vi "Close.vi"(8 "error in (no error)":errorcluster, 11 "State Variables in":T1={"NIVS.CachedDataRef"=refnum, "NIVS.LaunchRef"=refnum, "NIVS.SysDefRoot"=refnum, "NIVS.Workspace"=refnum, "NIVS.CachedData"={"Name"="", "Node Path"="", "Caption"="", "List"={"AutoUpdate"=FALSE, "Names"=[], "Values"=[], "Symbols"=[]}}, "NIVS.SystemStateRefs"={"CustDatRef"=refnum, "EvtRef"=refnum, "Target State User Event"=refnum}, "NIVS.UserEventRefs"={"SystemChangeEventRef"=refnum, "Event Registration Refnum"=refnum}, "Workspace.Connected?"=FALSE, "Workspace.ChannelFound?"=FALSE, "UI.Listbox"=refnum, "VS.DisplayFilter"=7, "Force?"=FALSE} {"VS.DisplayFilter" items=["K_CHAN_R", "K_CHAN_W", "K_CHAN_RW", "K_CHAN_VOLT", "K_CHAN_FAULT", "K_ALL", "K_CUSTOM", "K_CHAN_R_VIS", "K_CHAN_W_VIS", "K_CHAN_RW_VIS", "K_CHAN_VOLT_VIS", "K_CHAN_FAULT_VIS"]}) -> ()   [LabVIEW 2015, in "Workspace.Obejct.Radio.lvlib"]
uses:
  Workspace.Obejct.Radio.lvlib
  Types/StateVariables.ctl
  <vilib>/NI Veristand/Display Template Support/Display Template Support.llb/enum_Display Template Handler Minimal To Workspace.ctl
  <vilib>/NI Veristand/Display Template Support/Display Template Support.llb/enum_Display Template Handler Minimal To Widget Msg.ctl
  NationalInstruments.VeriStand.SystemStorage
  <vilib>/NI Veristand/Execution/Workspace/WorkspaceAPI.ctl
  NationalInstruments.VeriStand.ClientAPI
  Types/SavedStateData.ctl
  Types/Config.ctl
  <vilib>/NI Veristand/Execution/Workspace/SystemStateEventRef.ctl
  <vilib>/NI Veristand/Execution/Workspace/Target State Info.ctl
  <vilib>/NI Veristand/Execution/Workspace/Target State.ctl
  <vilib>/NI Veristand/Execution/Workspace/SystemStateRegEventRef.ctl
  <vilib>/NI Veristand/Execution/Workspace/NI_VS Workspace ExecutionAPI.lvlib
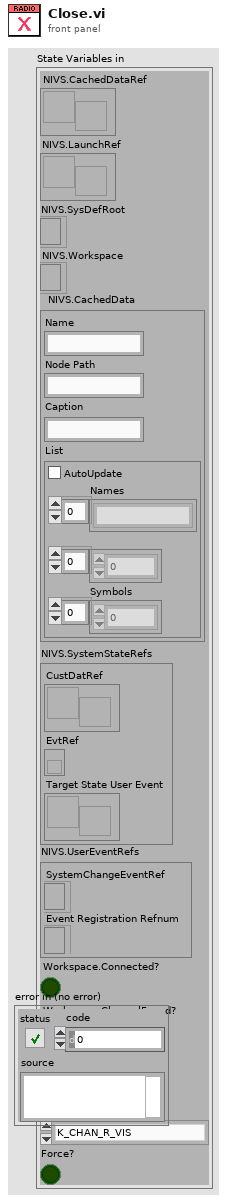
[diagram p1: front panel]
types:
  T1 = typedef "Workspace.Obejct.Radio.lvlib/StateVariables.ctl" = cluster{"NIVS.CachedDataRef":refnum<user-event>, "NIVS.LaunchRef":refnum<user-event>, "NIVS.SysDefRoot":refnum<k24>, "NIVS.Workspace":T2, "NIVS.CachedData":T3, "NIVS.SystemStateRefs":T5, "NIVS.UserEventRefs":cluster{"SystemChangeEventRef":T6, "Event Registration Refnum":refnum<event-registration>}, "Workspace.Connected?":bool, "Workspace.ChannelFound?":bool, "UI.Listbox":refnum<vi>, "VS.DisplayFilter":u8, "Force?":bool}
  T2 = typedef "NI_VS Workspace ExecutionAPI.lvlib/WorkspaceAPI.ctl" = refnum<k24>
  T3 = typedef "Workspace.Obejct.Radio.lvlib/SavedStateData.ctl" = cluster{"Name":string, "Node Path":string, "Caption":string, "List":T4}
  T4 = typedef "Workspace.Obejct.Radio.lvlib/Config.ctl" = cluster{"AutoUpdate":bool, "Names":string[], "Values":dbl[], "Symbols":i32[]}
  T5 = typedef "NI_VS Workspace ExecutionAPI.lvlib/SystemStateEventRef.ctl" = cluster{"CustDatRef":refnum<user-event>, "EvtRef":refnum<k27>, "Target State User Event":refnum<user-event>}
  T6 = typedef "NI_VS Workspace ExecutionAPI.lvlib/SystemStateRegEventRef.ctl" = refnum<event-registration>
  T7 = cluster{"SystemChangeEventRef":T6, "Event Registration Refnum":refnum<event-registration>}
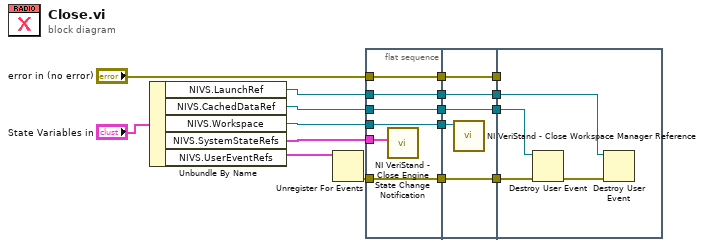
[diagram p0: block diagram]
diagram:
  n1 = Unbundle By Name("State Variables in") -> ("NIVS.LaunchRef"=w8:refnum<user-event>, "NIVS.CachedDataRef"=w7:refnum<user-event>, "NIVS.Workspace"=w6:T2, "NIVS.SystemStateRefs"=w5:T5, "NIVS.UserEventRefs"=w4:T7)
  n2 = Unregister For Events(event registration refnum=w4) -> (error out=w2:errorcluster)  [unwired: 1 in]
  n3 = flat-sequence {
    tunnel: w7 -> [w20]
    tunnel: w8 -> [w21]
    tunnel: w2 -> [w22]
    tunnel: "error in (no error)" -> [w23]
    tunnel: [w23] -> w17
    tunnel: [w22] -> w16
    tunnel: [w21] -> w15
    tunnel: [w20] -> w14
    tunnel: w5 -> [w19]
    tunnel: w6 -> [w18]
    tunnel: [w18] -> w13
    tunnel: w17 -> [w28]
    tunnel: [w28] -> w12
    tunnel: w16 -> [w27]
    tunnel: [w27] -> w11
    tunnel: w15 -> [w26]
    tunnel: [w26] -> w10
    tunnel: w14 -> [w25]
    tunnel: [w25] -> w9
    tunnel: w13 -> [w24]
    tunnel: w12 -> [_]
    tunnel: w11 -> [w30]
    tunnel: w10 -> [w32]
    tunnel: w9 -> [w31]
    frame #0 {
      n4 = call <vilib>:"NI VeriStand - Close Engine State Change Notification.vi"("SystemStateRefs"=w19) -> ()  [unwired: 10 in, 1 out]
    }
    frame #1 {
      n5 = call <vilib>:"NI VeriStand - Close Workspace Manager Reference.vi"("WorkspaceManager"=w24) -> ()  [unwired: 10 in, 1 out]
    }
    frame #2 {
      n6 = Destroy User Event(user event=w31, error in=w30) -> (error out=w29:errorcluster)
      n7 = Destroy User Event(user event=w32, error in=w29) -> ()  [unwired: 1 out]
    }
  }
